vi "Wait On Channel Value Change.vi"(8 "error in (no error)":errorcluster, 9 "Time to Wait":dbl caption="Time Target (s)", 10 "Channel":string, 11 ".NET Refnum in":T1) -> (0 "error out":errorcluster, 3 "Value":dbl)   [LabVIEW 2020, in "FPGA Addon DMA Waveform Status Channel System Tests.lvclass"]
uses:
  FPGA Addon DMA Waveform Status Channel System Tests.lvclass
  FPGA Addon DMA Waveform Status Channel System Tests.lvclass/FPGA Addon DMA Waveform Status Channel System Tests.ctl
  <vilib>/NI VeriStand/Execution/Workspace/NI_VS Workspace ExecutionAPI.lvlib
  <vilib>/NI VeriStand/Execution/Workspace/NI VeriStand - Get Single Channel Value.vi
  <vilib>/NI VeriStand/Execution/Workspace/WorkspaceAPI.ctl
  NationalInstruments.VeriStand.ClientAPI
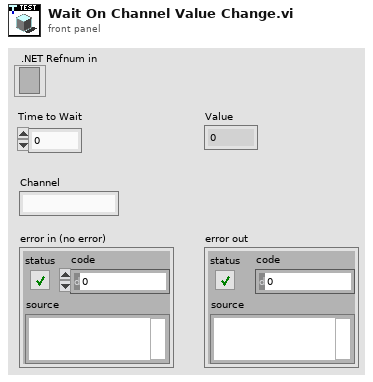
[diagram p1: front panel]
types:
  T1 = typedef "NI_VS Workspace ExecutionAPI.lvlib/WorkspaceAPI.ctl" = refnum<k24>
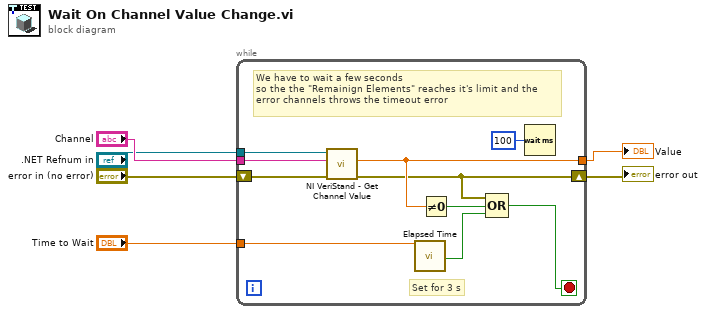
[diagram p0: block diagram]
diagram:
  n1 = while {
    shift-right: [w9] -> w4
    shift-left: "error in (no error)" -> [w16]
    tunnel: [w14] -> w6
    tunnel: ".NET Refnum in" -> [w15]
    tunnel: "Channel" -> [w8]
    tunnel: "Time to Wait" -> [w7]
    stop <- w12 stop-if-true
    # "Set for 3 s"
    # "We have to wait a few seconds \nso the the \"Remainign Elements\" reaches it's limit and the\nerror channels throws the timeout error"
    n2 = call-poly <vilib>:"NI VeriStand - Get Channel Value.vi"("error in (no error)"=w16, "Channel"=w8, "WorkspaceManager in"=w15) -> ("error out"=w9:errorcluster, "Value"=w14:dbl)  [unwired: 6 in, 1 out]
    n3 = call "Elapsed Time"("Time Target (s)"=w7) -> ("Time has Elapsed"=w11:bool)  [unwired: 11 in, 7 out]
    n4 = Not Equal To 0?(x=w14) -> (x != 0?=w13:bool)
    n5 = Compound Arithmetic op=OR(w9, w13, w11) -> (w12:bool)
    n6 = Wait (ms)(milliseconds to wait=u32 100) -> ()  [unwired: 1 out]
  }
  "Value" <- w6
  "error out" <- w4
